vi "Stop Channel.vi"(8 "error in (no error)":errorcluster, 11 "Potentiostat Galvanostat in":refnum<class "Potentiostat Galvanostat.lvclass">) -> (0 "error out":errorcluster, 3 "Potentiostat Galvanostat out":refnum<class "Potentiostat Galvanostat.lvclass">)   [LabVIEW 2018, in "Potentiostat Galvanostat.lvclass"]
uses:
  Potentiostat Galvanostat.lvclass
  Potentiostat Galvanostat.lvclass/Potentiostat Galvanostat.ctl
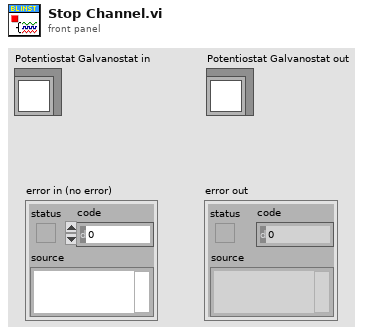
[diagram p1: front panel]
types:
  T1 = typedef "Potentiostat Galvanostat.lvclass/Channel.ctl" = u8
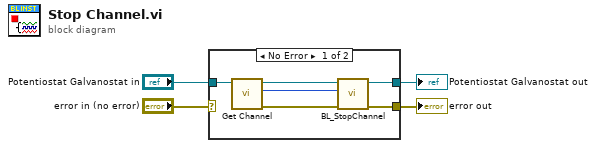
[diagram p0: block diagram]
diagram:
  n1 = case shown="No Error" "error in (no error)" {
    selector: "error in (no error)" -> [_ w12]
    tunnel: [w9 w12] -> w3
    tunnel: [w10 w11] -> w1
    tunnel: "Potentiostat Galvanostat in" -> [w8 w11]
    frame No Error {
      n2 = call "Get Channel.vi"("Potentiostat Galvanostat in"=w8) -> ("error out"=w6:errorcluster, "Channel"=w5:T1, "Potentiostat Galvanostat out"=w7:refnum<class "Potentiostat Galvanostat.lvclass">)  [unwired: 8 in]
      n3 = call "BL_StopChannel.vi"("error in (no error)"=w6, "Channel"=w5, "Potentiostat Galvanostat in"=w7) -> ("error out"=w9:errorcluster, "Potentiostat Galvanostat out"=w10:refnum<class "Potentiostat Galvanostat.lvclass">)  [unwired: 6 in, 1 out]
    }
    frame Error {
    }
  }
  "error out" <- w3
  "Potentiostat Galvanostat out" <- w1
